vi "Release Lines Points.vi"(8 "error in (no error)":errorcluster, 10 "Auto Release  Line Points":T1={"Auto Release Points 1 X (enabled)"=FALSE, "Auto Release Points 1 Y (enabled)"=FALSE, "Auto Release Points 2 X (enabled)"=FALSE, "Auto Release Points 2 Y (enabled)"=FALSE, "Auto Release Keys (enabled)"=TRUE}, 11 "Lines":T2) -> (0 "error out":errorcluster)   [LabVIEW 2020, in "G2CPU Line Profile.lvlib"]
uses:
  G2CPU Line Profile.lvlib
  <vilib>/Natan Biesmans/G2CPU GPU and CPU HPC Toolkit/G2CPU Libraries/Arrays/1DArray/f32/1D Array f32.lvclass
  C:/Program Files/National Instruments/LabVIEW 2025/vi.lib/Natan Biesmans/G2CPU GPU and CPU HPC Toolkit/G2CPU Libraries/Arrays/Array/Array Prototype.lvclass
  <vilib>/Natan Biesmans/G2CPU GPU and CPU HPC Toolkit/G2CPU Libraries/Arrays/1DArray/u32/1D Array u32.lvclass
  <vilib>/Natan Biesmans/G2CPU GPU and CPU HPC Toolkit/G2CPU Libraries/Arrays/Array/Array Prototype.lvclass
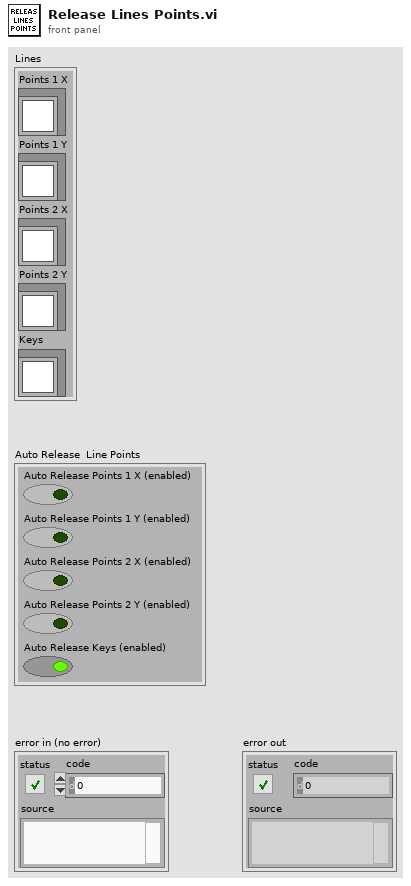
[diagram p1: front panel]
types:
  T1 = cluster{"Auto Release Points 1 X (enabled)":bool, "Auto Release Points 1 Y (enabled)":bool, "Auto Release Points 2 X (enabled)":bool, "Auto Release Points 2 Y (enabled)":bool, "Auto Release Keys (enabled)":bool}
  T2 = cluster{"Points 1 X":refnum<class "1D Array f32.lvclass">, "Points 1 Y":refnum<class "1D Array f32.lvclass">, "Points 2 X":refnum<class "1D Array f32.lvclass">, "Points 2 Y":refnum<class "1D Array f32.lvclass">, "Keys":refnum<class "1D Array u32.lvclass">}
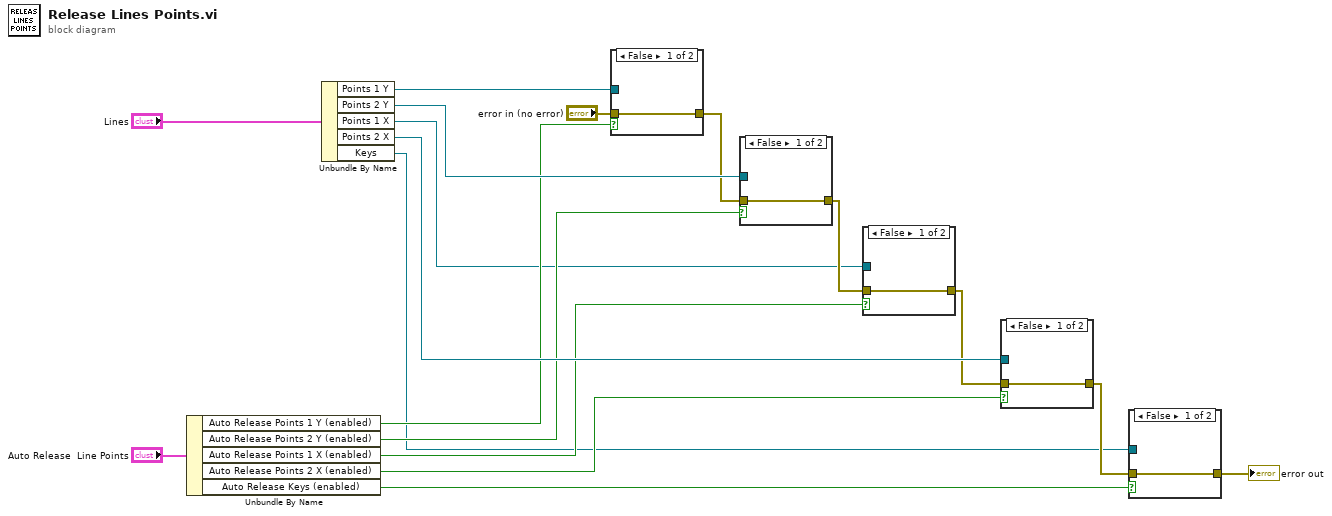
[diagram p0: block diagram]
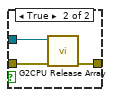
[diagram p2: hidden frame]
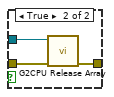
[diagram p3: hidden frame]
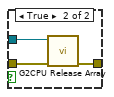
[diagram p4: hidden frame]
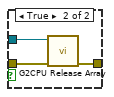
[diagram p5: hidden frame]
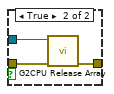
[diagram p6: hidden frame]
diagram:
  n1 = Unbundle By Name("Auto Release  Line Points") -> ("Auto Release Points 1 Y (enabled)"=w11:bool, "Auto Release Points 2 Y (enabled)"=w12:bool, "Auto Release Points 1 X (enabled)"=w13:bool, "Auto Release Points 2 X (enabled)"=w14:bool, "Auto Release Keys (enabled)"=w3:bool)
  n2 = Unbundle By Name("Lines") -> ("Points 1 Y"=w18:refnum<class "1D Array f32.lvclass">, "Points 2 Y"=w17:refnum<class "1D Array f32.lvclass">, "Points 1 X"=w1:refnum<class "1D Array f32.lvclass">, "Points 2 X"=w16:refnum<class "1D Array f32.lvclass">, "Keys"=w4:refnum<class "1D Array u32.lvclass">)
  n3 = case shown="False" w11 {
    tunnel: w18 -> [_ w21]
    tunnel: "error in (no error)" -> [w19 w22]
    tunnel: [w19 w20] -> w7
    frame False {
    }
    frame True {
      n4 = call <vilib>:"G2CPU Release Array.vi"("error in (no error)"=w22, "Array in"=w21) -> ("error out"=w20:errorcluster)  [unwired: 9 in]
    }
  }
  n5 = case shown="False" w12 {
    tunnel: w17 -> [_ w25]
    tunnel: w7 -> [w23 w26]
    tunnel: [w23 w24] -> w8
    frame False {
    }
    frame True {
      n6 = call <vilib>:"G2CPU Release Array.vi"("error in (no error)"=w26, "Array in"=w25) -> ("error out"=w24:errorcluster)  [unwired: 9 in]
    }
  }
  n7 = case shown="False" w13 {
    tunnel: w1 -> [_ w29]
    tunnel: w8 -> [w27 w30]
    tunnel: [w27 w28] -> w9
    frame False {
    }
    frame True {
      n8 = call <vilib>:"G2CPU Release Array.vi"("error in (no error)"=w30, "Array in"=w29) -> ("error out"=w28:errorcluster)  [unwired: 9 in]
    }
  }
  n9 = case shown="False" w14 {
    tunnel: w16 -> [_ w33]
    tunnel: w9 -> [w31 w34]
    tunnel: [w31 w32] -> w5
    frame False {
    }
    frame True {
      n10 = call <vilib>:"G2CPU Release Array.vi"("error in (no error)"=w34, "Array in"=w33) -> ("error out"=w32:errorcluster)  [unwired: 9 in]
    }
  }
  n11 = case shown="False" w3 {
    tunnel: w4 -> [_ w37]
    tunnel: w5 -> [w35 w38]
    tunnel: [w35 w36] -> w2
    frame False {
    }
    frame True {
      n12 = call <vilib>:"G2CPU Release Array.vi"("error in (no error)"=w38, "Array in"=w37) -> ("error out"=w36:errorcluster)  [unwired: 9 in]
    }
  }
  "error out" <- w2
